vi "loadDataNodeBegin.vi"(8 "error in (no error)":errorcluster, 10 "XML Refnum in":refnum<file>, 11 "Channel in":refnum<class "Channel.lvclass">) -> (0 "error out":errorcluster, 2 "XML Refnum out":refnum<file>, 3 "Channel out":refnum<class "Channel.lvclass">)   [LabVIEW 2014, in "Channel.lvclass"]
doc: "Part of the file loading process. Occurs at the beginning of a node being loaded. Loads the common xceDataNode data name and description."
uses:
  Channel.lvclass
  Channel.lvclass/Channel.ctl
  xCE/xceDataNode/xceDataNode.lvclass
  XML Parser/XML Parser.lvclass
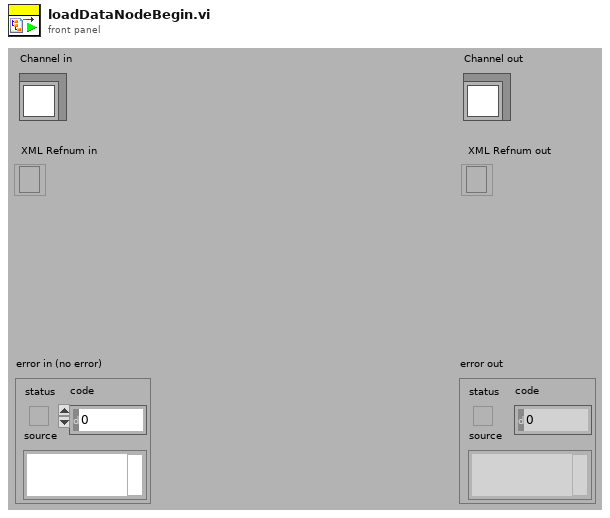
[diagram p1: front panel]
types:
  T1 = typedef "enum_Symbols.ctl" = enum16{"Default", "Analog Input", "Analog Output", "Digital Input", "Digital Output", "PWM Input", "PWM Output"}
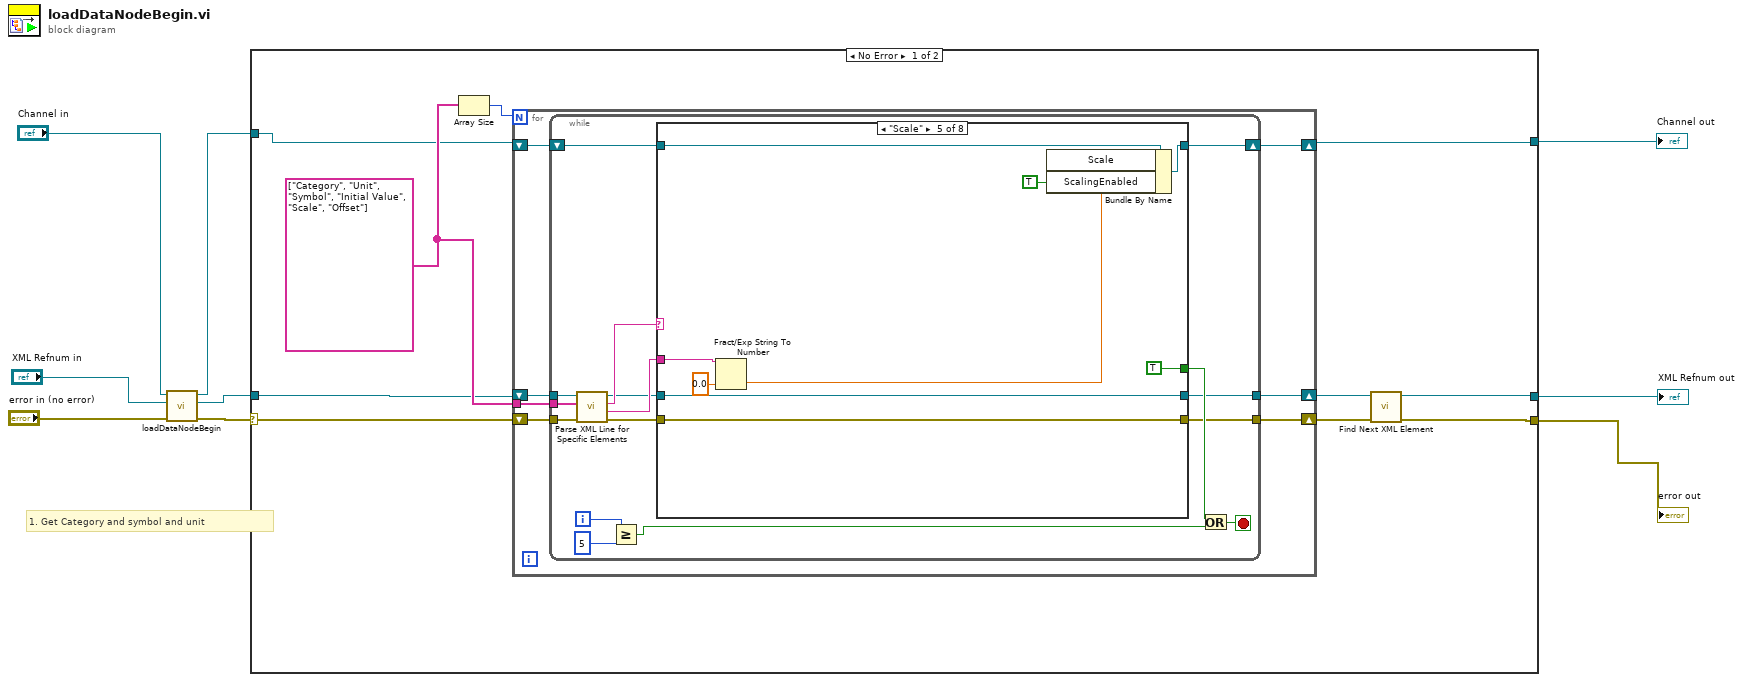
[diagram p0: block diagram]
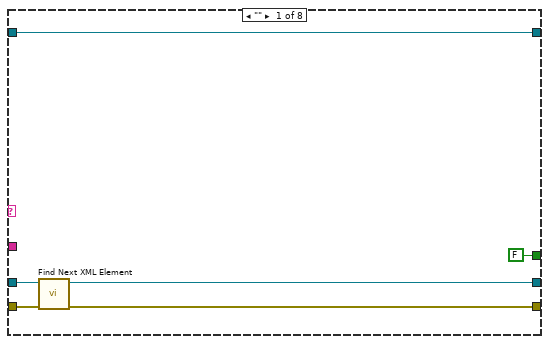
[diagram p2: hidden frame]
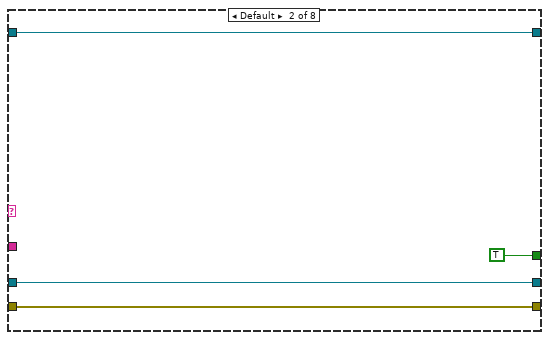
[diagram p3: hidden frame]
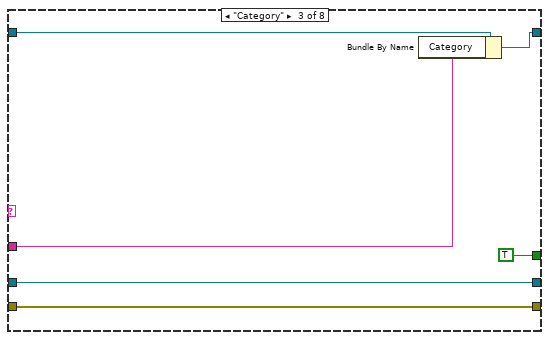
[diagram p4: hidden frame]
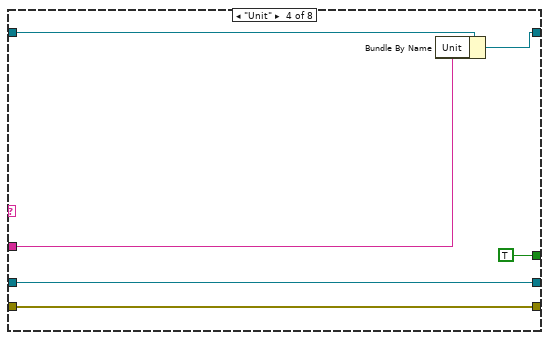
[diagram p5: hidden frame]
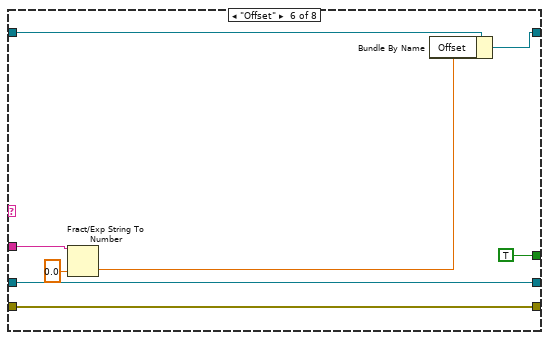
[diagram p6: hidden frame]
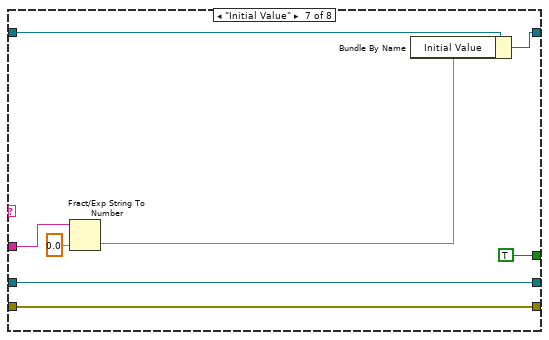
[diagram p7: hidden frame]
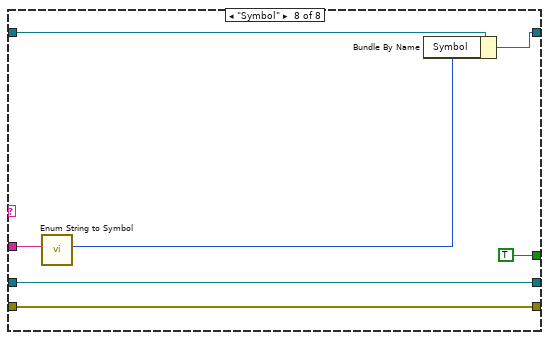
[diagram p8: hidden frame]
diagram:
  # "1. Get Category and symbol and unit"
  n1 = call-parent "loadDataNodeBegin.vi"("error in (no error)"="error in (no error)", "XML Refnum in"="XML Refnum in", "xceDataNode in"="Channel in") -> ("error out"=w6:errorcluster, "XML Refnum out"=w3:refnum<file>, "xceDataNode out"=w1:refnum<class "Channel.lvclass">)  [unwired: 6 in]
  n2 = case shown="No Error" w6 {
    selector: w6 -> [w15 w99]
    tunnel: [w11 w99] -> w7
    tunnel: [w14 w97] -> w9
    tunnel: w3 -> [w16 w98]
    tunnel: [w10 w98] -> w8
    tunnel: w1 -> [w17 w97]
    frame No Error {
      w18 = string[] ["Category", "Unit", "Symbol", "Initial Value", "Scale", "Offset"] ("Token List")
      n3 = Array Size(array=w18) -> (size(s)=w19:i32)
      n4 = for {
        N: w19 -> [_]
        tunnel: w18 -> [w26]
        shift-right: [w21] -> w14
        shift-left: w17 -> [w23]
        shift-right: [w22] -> w13
        shift-left: w16 -> [w25]
        shift-right: [w20] -> w12
        shift-left: w15 -> [w24]
        n5 = while {
          tunnel: w26 -> [w42]
          tunnel: w25 -> [w41]
          tunnel: w24 -> [w40]
          shift-right: [w35] -> w21
          shift-left: w23 -> [w37]
          tunnel: [w27] -> w22
          tunnel: [w28] -> w20
          i -> [w39]
          stop <- w32 stop-if-true
          n6 = call "Parse XML Line for Specific Elements.vi"("error in (no error)"=w40, "Elements"=w42, "XML Refnum in"=w41) -> ("error out"=w29:errorcluster, "Value"=w31:string, "Element Name"=w36:string, "XML Refnum out"=w30:refnum<file>)  [unwired: 4 in, 1 out]
          n7 = Greater Or Equal?(x=w39, y=5) -> (x >= y?=w33:bool)
          n8 = case shown="\"Scale\"" w36 {
            tunnel: w37 -> [w48 w52 w58 w64 w73 w81 w89 w96]
            tunnel: [w48 w52 w57 w63 w72 w80 w88 w95] -> w35
            tunnel: [FALSE TRUE TRUE TRUE TRUE TRUE TRUE TRUE] -> w34
            tunnel: w31 -> [_ _ w53 w59 w67 w75 w83 w91]
            tunnel: w30 -> [w45 w50 w55 w61 w70 w78 w86 w93]
            tunnel: w29 -> [w46 w49 w54 w60 w69 w77 w85 w92]
            tunnel: [w43 w49 w54 w60 w69 w77 w85 w92] -> w28
            tunnel: [w44 w50 w55 w61 w70 w78 w86 w93] -> w27
            frame "" {
              n9 = call "Find Next XML Element.vi"("error in (no error)"=w46, "XML Fine In"=w45) -> ("error out"=w43:errorcluster, "XML Fine Out"=w44:refnum<file>)  [unwired: 7 in, 1 out]
            }
            frame Default {
            }
            frame "Category" {
              n10 = Bundle By Name(cluster=w58, "Category"=w53) -> (w57:refnum<class "Channel.lvclass">)
            }
            frame "Unit" {
              n11 = Bundle By Name(cluster=w64, "Unit"=w59) -> (w63:refnum<class "Channel.lvclass">)
            }
            frame "Scale" {
              n12 = Fract/Exp String To Number(string=w67, default (0 dbl)=0.0 ("default (0 DBL)")) -> (number=w66:dbl)  [unwired: 2 in, 1 out]
              n13 = Bundle By Name(cluster=w73, "Scale"=w66, "ScalingEnabled"=TRUE) -> (w72:refnum<class "Channel.lvclass">)
            }
            frame "Offset" {
              n14 = Fract/Exp String To Number(string=w75, default (0 dbl)=0.0 ("default (0 DBL)")) -> (number=w74:dbl)  [unwired: 2 in, 1 out]
              n15 = Bundle By Name(cluster=w81, "Offset"=w74) -> (w80:refnum<class "Channel.lvclass">)
            }
            frame "Initial Value" {
              n16 = Fract/Exp String To Number(string=w83, default (0 dbl)=0.0 ("default (0 DBL)")) -> (number=w82:dbl)  [unwired: 2 in, 1 out]
              n17 = Bundle By Name(cluster=w89, "Initial Value"=w82) -> (w88:refnum<class "Channel.lvclass">)
            }
            frame "Symbol" {
              n18 = call "Enum String to Symbol.vi"("Symbol String In"=w91) -> ("Symbol Enum Out"=w90:T1)  [unwired: 10 in]
              n19 = Bundle By Name(cluster=w96, "Symbol"=w90) -> (w95:refnum<class "Channel.lvclass">)
            }
          }
          n20 = Or(x=w34, y=w33) -> (x .or. y?=w32:bool)
        }
      }
      n21 = call "Find Next XML Element.vi"("error in (no error)"=w12, "XML Fine In"=w13) -> ("error out"=w11:errorcluster, "XML Fine Out"=w10:refnum<file>)  [unwired: 7 in, 1 out]
    }
    frame Error {
    }
  }
  "error out" <- w7
  "Channel out" <- w9
  "XML Refnum out" <- w8
